vi "Items.vi"(8 "error in (no error)":errorcluster, 11 "StringList in":refnum<class "StringList.lvclass">) -> (0 "error out":errorcluster, 1 "Strings":string[](array[string]), 3 "StringList out":refnum<class "StringList.lvclass">)   [LabVIEW 2013, in "LapDog.Collections.v_.Lists.lvlib" / "StringList.lvclass"]
uses:
  StringList.lvclass
  LapDog.Collections.Common/String/String.lvclass
  ObjectList/ObjectList.lvclass
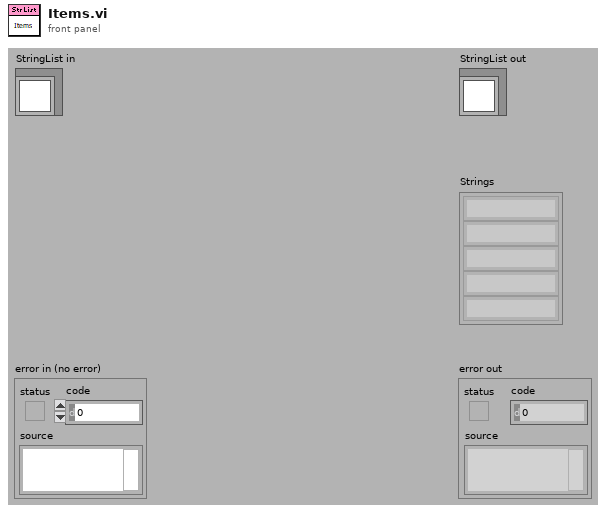
[diagram p1: front panel]
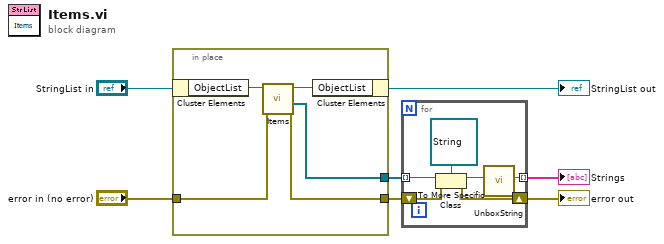
[diagram p0: block diagram]
diagram:
  n1 = in-place {
    in-place-border: "error in (no error)" -> [w10]
    in-place-border: [w9] -> w3
    in-place-border: [w8] -> w2
    n2 = in-place-cluster #1("StringList in") -> ("ObjectList"=w12:refnum<class "ObjectList.lvclass">)
    n3 = call-dynamic "Items.vi"("error in (no error)"=w10, "List in"=w12) -> ("error out"=w9:errorcluster, "Items"=w8:refnum<class>[], "List out"=w11:refnum<class "ObjectList.lvclass">)  [unwired: 7 in]
    n4 = in-place-cluster #1("ObjectList"=w11) -> (→"StringList out":refnum<class "StringList.lvclass">)
  }
  n5 = for {
    tunnel: w2 -> [w16] mode=indexing
    shift-right: [w18] -> w4
    shift-left: w3 -> [w17]
    tunnel: [w13] -> w1 mode=indexing
    n6 = To More Specific Class(target class=refnum<class "String.lvclass"> refnum ("LapDog.Collections.v0.Lists.Interfaces.lvlib:String.lvclass"), reference=w16, error in=w17) -> (specific class reference=w14:refnum<class "String.lvclass">, error out=w18:errorcluster)
    n7 = call "UnboxString.vi"("String in"=w14) -> ("String"=w13:string)  [unwired: 10 in]
  }
  "error out" <- w4
  "Strings" <- w1
